vi "wrap data.vi"(10 "identifier":string, 11 "data to wrap":string) -> (3 "wrapped data":string)   [LabVIEW 2025, in "CEF.lvlib" / "CEF_serializable configuration.lvclass"]
doc: "Generates a packed dataset of the form:\n<identifier>data to wrap</identifier>Copyright 2017 National Instruments Corporation\n\nLicensed under the Apache License, Version 2.0 (the \"License\"); you may not use this file except in compliance with the License. You may obtain a copy of the License at http://www.apache.org/licenses/LICENSE-2.0\nUnless required by applicable law or agreed to in writing, software distributed under the License is distributed on an \"AS IS\" BASIS, WITHOUT WARRANTIES OR CONDITIONS OF ANY KIND, either express or implied. See the License for the specific language governing permissions and limitations under the License."
uses:
  CEF_serializable configuration.lvclass
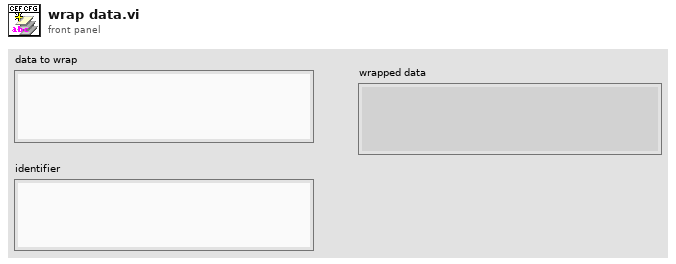
[diagram p1: front panel]
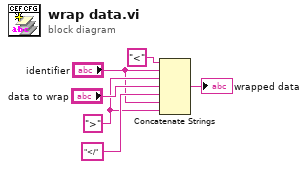
[diagram p0: block diagram]
diagram:
  w2 = ">" ("string")
  n1 = Concatenate Strings("<" ("string"), "identifier", w2, "data to wrap", "</" ("string"), "identifier", w2) -> (→"wrapped data":string)
